vi "SetSlideSpeed.vi"(8 "error in (no error)":errorcluster, 10 "Speed_x":dbl) -> (0 "error out":errorcluster)   [LabVIEW 2019, in "RT_Game.lvlib" / "Engine.lvclass"]
uses:
  Engine.lvclass
  MessageCluster.ctl
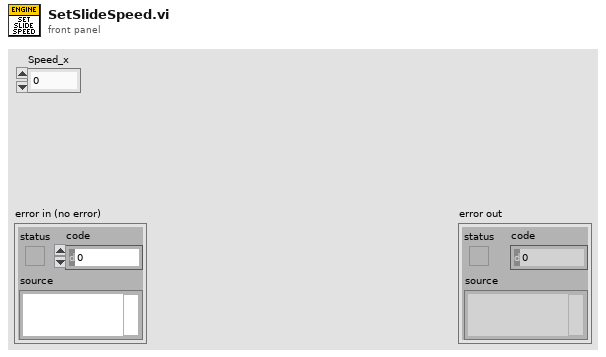
[diagram p1: front panel]
types:
  T1 = typedef "RT_Game.lvlib/Engine.lvclass/MessageCluster.ctl" = cluster{"Message":string, "Data":variant}
  T2 = typedef "RT_Game.lvlib/Engine.lvclass/Queues.ctl" = cluster{"MusicQueue":refnum<queue>, "TilesQueue":refnum<queue>, "SoundsQueue":refnum<queue>}
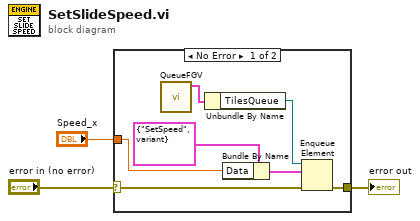
[diagram p0: block diagram]
diagram:
  n1 = case shown="No Error" "error in (no error)" {
    selector: "error in (no error)" -> [w10 w11]
    tunnel: [w9 w11] -> w2
    tunnel: "Speed_x" -> [w6 _]
    frame No Error {
      n2 = call "QueueFGV.vi"() -> ("Queues out"=w5:T2)  [unwired: 10 in, 1 out]
      n3 = Unbundle By Name(w5) -> ("TilesQueue"=w4:refnum<queue>)
      n4 = Bundle By Name(cluster=T1 {"Message"="SetSpeed", "Data"=variant} ("element"), "Data"=w6) -> (w7:T1)
      n5 = Enqueue Element(queue=w4, element=w7, error in (no error)=w10) -> (error out=w9:errorcluster)  [unwired: 1 in, 2 out]
    }
    frame Error {
    }
  }
  "error out" <- w2
